vi "SetAxisNumericParameter(Int).vi"(7 "CMD":string, 8 "error in (no error)":errorcluster, 9 "ParameterValue":i32, 11 "Picomoto8742ControllerClass in":refnum<class "Picomoto8742ControllerClass.lvclass">) -> (0 "error out":errorcluster, 3 "Picomoto8742ControllerClass Out":refnum<class "Picomoto8742ControllerClass.lvclass">)   [LabVIEW 2013, in "Picomoto8742ControllerClass.lvclass"]
doc: "Send a numeric parameter (Int32) command to the physical device"
uses:
  Picomoto8742ControllerClass.lvclass
  Picomoto8742ControllerClass.lvclass/Picomoto8742ControllerClass.ctl
  PicoMotor8472Comm/PicoMotor8742Comm.lvclass
  PicoMotor8742Axis/Picomotor8742Axis.lvclass
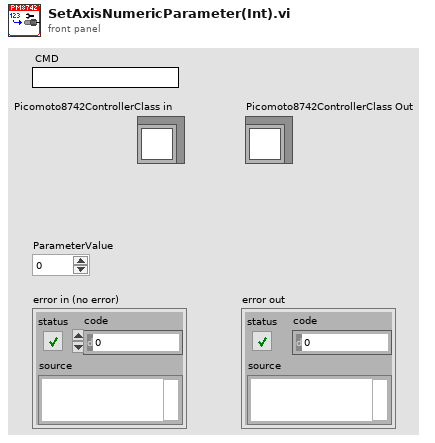
[diagram p1: front panel]
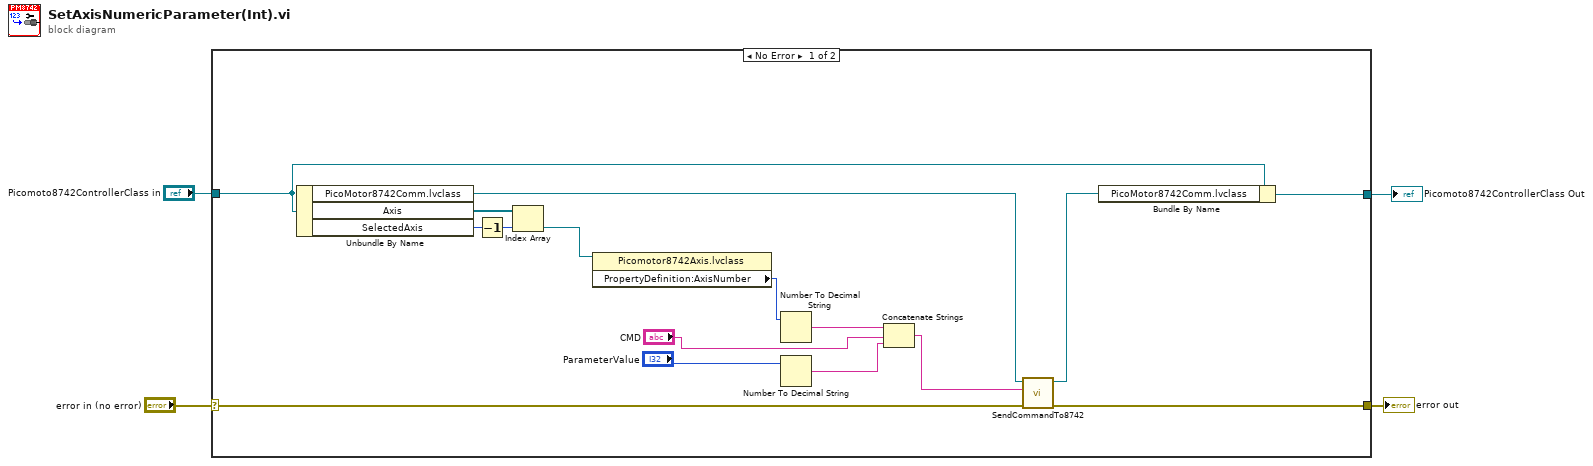
[diagram p0: block diagram]
diagram:
  n1 = case shown="No Error" "error in (no error)" {
    selector: "error in (no error)" -> [w15 w22]
    tunnel: [w14 w22] -> w4
    tunnel: "Picomoto8742ControllerClass in" -> [w9 w21]
    tunnel: [w12 w21] -> w1
    frame No Error {
      n2 = Unbundle By Name(w9) -> ("PicoMotor8742Comm.lvclass"=w7:refnum<class "PicoMotor8742Comm.lvclass">, "Axis"=w10:refnum<class "Picomotor8742Axis.lvclass">[], "SelectedAxis"=w6:u32)
      n3 = Decrement(x=w6) -> (x-1=w5:u32)
      n4 = Index Array(array=w10, index=w5) -> (element=w11:refnum<class "Picomotor8742Axis.lvclass">)
      n5 = property class="Picomotor8742Axis.lvclass"(reference=w11) -> ("PropertyDefinition:AxisNumber"=w8:i32)  [unwired: 1 in, 2 out]
      n6 = Number To Decimal String(number=w8) -> (decimal integer string=w18:string)  [unwired: 1 in]
      n7 = Number To Decimal String(number="ParameterValue") -> (decimal integer string=w20:string)  [unwired: 1 in]
      n8 = Concatenate Strings(w18, "CMD", w20) -> (w16:string)
      n9 = call-dynamic "SendCommandTo8742.vi"("error in (no error)"=w15, "Command"=w16, "PicoMotor8742Comm in"=w7) -> ("error out"=w14:errorcluster, "PicoMotor8742Comm out"=w13:refnum<class "PicoMotor8742Comm.lvclass">)  [unwired: 6 in, 1 out]
      n10 = Bundle By Name(cluster=w9, "PicoMotor8742Comm.lvclass"=w13) -> (w12:refnum<class "Picomoto8742ControllerClass.lvclass">)
    }
    frame Error {
    }
  }
  "error out" <- w4
  "Picomoto8742ControllerClass Out" <- w1
